vi "Open SequenceFile.vi"(8 "error in (no error)":errorcluster, 10 "File Load Options":T1={"Use Search Dirs? (T)"=TRUE, "Conflict as Error? (T)"=TRUE, "Check Station Model? (F)"=FALSE, "Preload Modules? (T)"=TRUE, "Skip Load Callback? (F)"=FALSE, "Reload if Loaded? (F)"=FALSE}, 11 "Path":path) -> (0 "error out":errorcluster, 3 "SequenceFile out":refnum<class "SequenceFile.lvclass">)   [LabVIEW 2020, in "TSnax.lvlib" / "SequenceFile.lvclass"]
uses:
  SequenceFile.lvclass
  SequenceFile.lvclass/SequenceFile.ctl
  Engine/Engine.lvclass
  File Load Options.ctl
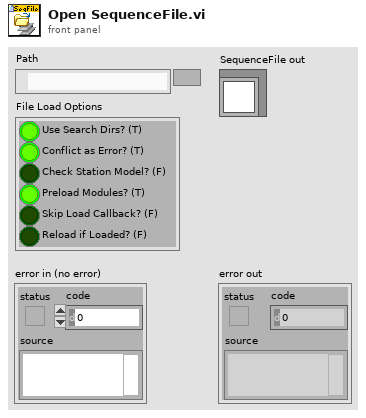
[diagram p1: front panel]
types:
  T1 = typedef "TSnax.lvlib/SequenceFile.lvclass/File Load Options.ctl" = cluster{"Use Search Dirs? (T)":bool, "Conflict as Error? (T)":bool, "Check Station Model? (F)":bool, "Preload Modules? (T)":bool, "Skip Load Callback? (F)":bool, "Reload if Loaded? (F)":bool}
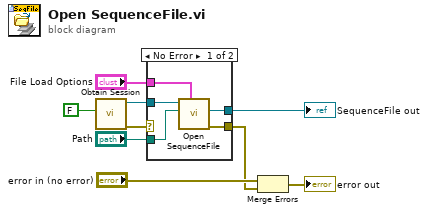
[diagram p0: block diagram]
diagram:
  n1 = call "Obtain Session.vi"("Create if needed? (T)"=FALSE) -> ("error out"=w6:errorcluster, "Engine out"=w7:refnum<class "Engine.lvclass">)  [unwired: 9 in]
  n2 = case shown="No Error" w6 {
    selector: w6 -> [_ w15]
    tunnel: w7 -> [w14 _]
    tunnel: "Path" -> [w13 _]
    tunnel: "File Load Options" -> [w12 _]
    tunnel: [w11 _] -> w3
    tunnel: [w10 w15] -> w1
    frame No Error {
      n3 = call "Open SequenceFile.vi"("File Load Options"=w12, "File Path"=w13, "Engine in"=w14) -> ("error out"=w10:errorcluster, "SequenceFile"=w11:refnum<class "SequenceFile.lvclass">)  [unwired: 6 in, 1 out]
    }
    frame Error {
    }
  }
  "SequenceFile out" <- w3
  n4 = Merge Errors("error in (no error)", w1) -> (→"error out":errorcluster)
